vi "parse_error_response.vi"(0 "headers":string, 5 "body":string, 11 "error in (no error)":errorcluster) -> (4 "error messages":string, 15 "error out":errorcluster)   [LabVIEW 2020, in "vector_weviate.lvclass"]
doc: "This VI parses the error response"
uses:
  vector_weviate.lvclass
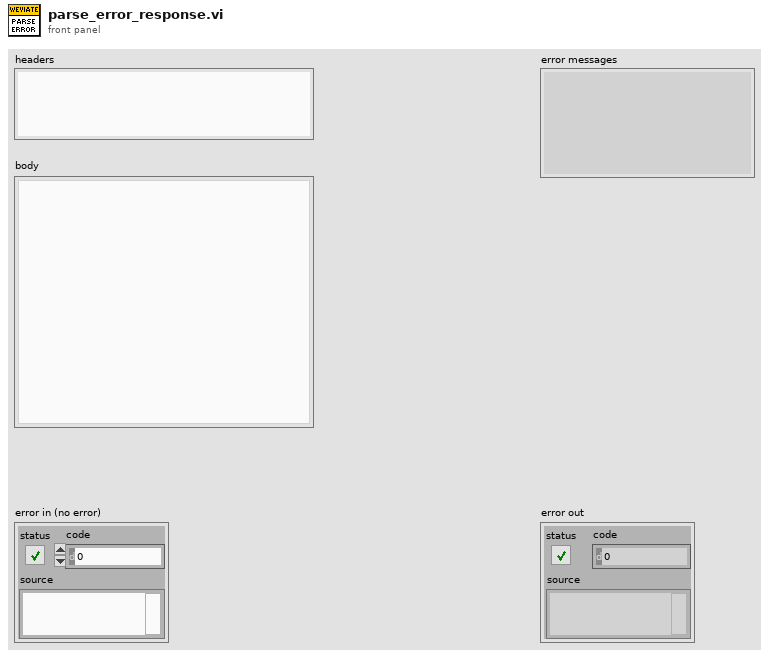
[diagram p1: front panel]
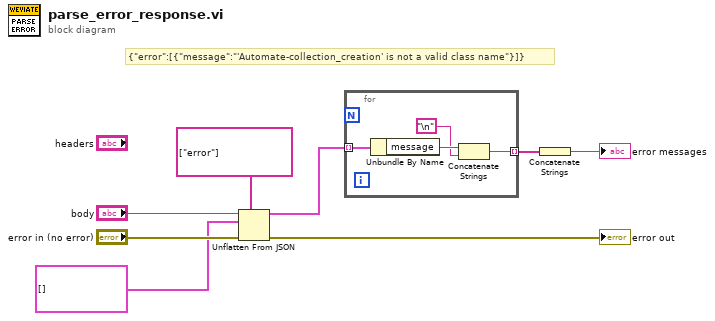
[diagram p0: block diagram]
diagram:
  # "{\"error\":[{\"message\":\"'Automate-collection_creation' is not a valid class name\"}]}"
  n1 = Unflatten From JSON(path=string[] ["error"], JSON string="body", type and defaults=cluster{"message":string}[] [], error in (no error)="error in (no error)") -> (value=w4:cluster{"message":string}[], error out=→"error out":errorcluster)  [unwired: 3 in]
  n2 = for {
    tunnel: w4 -> [w12] mode=indexing
    tunnel: [w10] -> w2 mode=indexing
    n3 = Unbundle By Name(w12) -> ("message"=w11:string)
    n4 = Concatenate Strings(w11, "\n") -> (w10:string)
  }
  n5 = Concatenate Strings(w2) -> (→"error messages":string)
